vi "write_conditions_to_scope.vi"(0 "instrument handle":refnum<k15> caption="instrument handle in", 1 "Controls Cluster In":T4={"Scope Channel"="", "C1 vertical offset / V"=0.0, "C1 vertical range / V"=5.0, "C1 probe attenuation"=1.0, "C1 vertical coupling / V"=1, "C1 enabled"=TRUE, "C1 maximum input frequency / Hz"=0.0, "C1 input impedance / ohms"=0, "C2 vertical offset / V"=0.0, "C2 vertical range / V"=5.0, "C2 probe attenuation"=1.0, "C2 vertical coupling / V"=1, "C2 enabled"=TRUE, "C2 maximum input frequency / Hz"=0.0, "C2 input impedance / ohms"=0, "Enforce realtime"=TRUE, "Samples"=0, "tmax / us "=0.0, "Trigger source"="0", "Trigger slope"=0, "Trigger delay / us"=0.0} {"C1 vertical coupling / V" items=["AC", "DC", "Ground"]; "C1 input impedance / ohms" items=["1 mega ohm"=0, "50 ohms"=2]; "C2 vertical coupling / V" items=["AC", "DC", "Ground"]; "C2 input impedance / ohms" items=["1 mega ohm"=0, "50 ohms"=2]; "Samples" items=["500 S"=500, "1 kS"=1000, "5 kS"=5000, "10 kS"=10000, "100 kS"=100000, "500 kS"=500000, "1 MS"=1000000, "2.5 MS"=2500000, "5MS"=5000000, "10 MS"=10000000, "20 MS"=20000000]; "Trigger slope" items=["Positive", "Negative"]}, 11 "error in":errorcluster) -> (3 "Controls Cluster Out":T4={"Scope Channel"="", "C1 vertical offset / V"=0.0, "C1 vertical range / V"=5.0, "C1 probe attenuation"=1.0, "C1 vertical coupling / V"=1, "C1 enabled"=TRUE, "C1 maximum input frequency / Hz"=0.0, "C1 input impedance / ohms"=0, "C2 vertical offset / V"=0.0, "C2 vertical range / V"=5.0, "C2 probe attenuation"=1.0, "C2 vertical coupling / V"=1, "C2 enabled"=TRUE, "C2 maximum input frequency / Hz"=0.0, "C2 input impedance / ohms"=0, "Enforce realtime"=TRUE, "Samples"=0, "tmax / us "=0.0, "Trigger source"="0", "Trigger slope"=0, "Trigger delay / us"=0.0} {"C1 vertical coupling / V" items=["AC", "DC", "Ground"]; "C1 input impedance / ohms" items=["1 mega ohm"=0, "50 ohms"=2]; "C2 vertical coupling / V" items=["AC", "DC", "Ground"]; "C2 input impedance / ohms" items=["1 mega ohm"=0, "50 ohms"=2]; "Samples" items=["500 S"=500, "1 kS"=1000, "5 kS"=5000, "10 kS"=10000, "100 kS"=100000, "500 kS"=500000, "1 MS"=1000000, "2.5 MS"=2500000, "5MS"=5000000, "10 MS"=10000000, "20 MS"=20000000]; "Trigger slope" items=["Positive", "Negative"]}, 4 "instrument handle out":refnum<k15>, 15 "error out":errorcluster)   [LabVIEW 2023]
uses:
  <instrlib>/niScope/Controls/niScope vertical coupling.ctl
  <instrlib>/niScope/Controls/niScope trigger source.ctl
  <instrlib>/niScope/Controls/niScope trigger slope.ctl
  <instrlib>/niScope/Configure/Trigger/niScope Configure Trigger Digital.vi
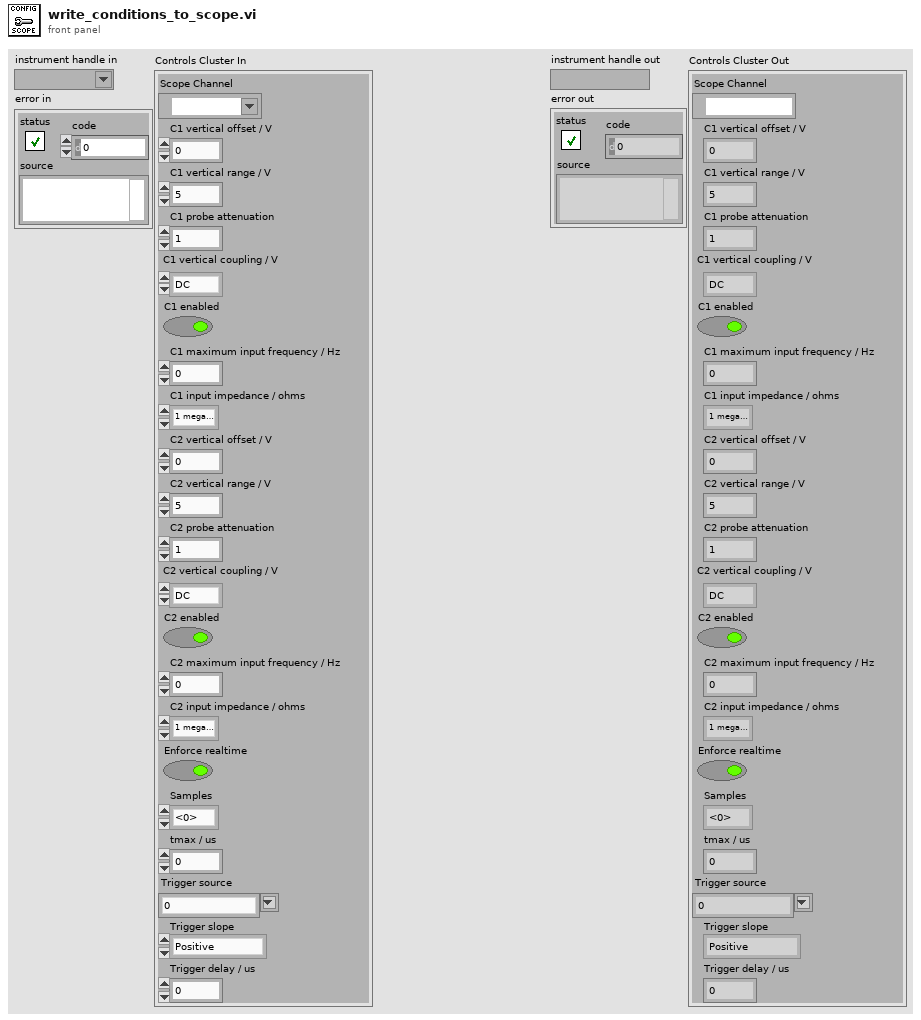
[diagram p1: front panel]
types:
  T1 = typedef "niScope vertical coupling.ctl" = i32
  T2 = typedef "niScope trigger source.ctl" = string
  T3 = typedef "niScope trigger slope.ctl" = i32
  T4 = cluster{"Scope Channel":refnum<k15>, "C1 vertical offset / V":dbl, "C1 vertical range / V":dbl, "C1 probe attenuation":dbl, "C1 vertical coupling / V":T1, "C1 enabled":bool, "C1 maximum input frequency / Hz":dbl, "C1 input impedance / ohms":u32, "C2 vertical offset / V":dbl, "C2 vertical range / V":dbl, "C2 probe attenuation":dbl, "C2 vertical coupling / V":T1, "C2 enabled":bool, "C2 maximum input frequency / Hz":dbl, "C2 input impedance / ohms":u32, "Enforce realtime":bool, "Samples":i64, "tmax / us ":dbl, "Trigger source":T2, "Trigger slope":T3, "Trigger delay / us":dbl}
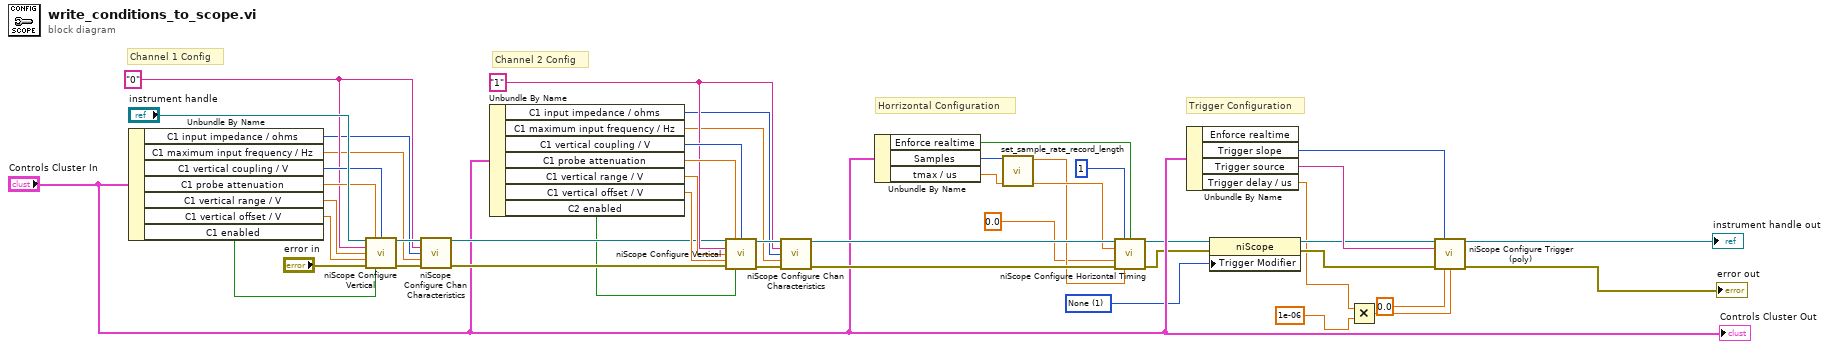
[diagram p0: block diagram]
diagram:
  w4 = 1 items=["None"=1, "Auto Trigger"=2] ("Triggering:Trigger Modifier")
  w30 = "1" ("channels")
  w39 = "0" ("channels")
  # "Trigger Configuration"
  # "Channel 2 Config"
  # "Horrizontal Configuration"
  # "Channel 1 Config"
  n1 = Unbundle By Name("Controls Cluster In") -> ("C1 input impedance / ohms"=w35:u32, "C1 maximum input frequency / Hz"=w36:dbl, "C1 vertical coupling / V"=w40:T1, "C1 probe attenuation"=w41:dbl, "C1 vertical range / V"=w38:dbl, "C1 vertical offset / V"=w37:dbl, "C1 enabled"=w12:bool)
  n2 = call <instrlib>:"niScope Configure Vertical.vi"("instrument handle"="instrument handle", "probe attenuation"=w41, "vertical coupling"=w40, "channels"=w39, "vertical range"=w38, "vertical offset"=w37, "error in"="error in", "channel enabled"=w12) -> ("instrument handle out"=w47:refnum<k15>, "error out"=w46:errorcluster)  [unwired: 6 in]
  n3 = call <instrlib>:"niScope Configure Chan Characteristics.vi"("instrument handle"=w47, "channels"=w39, "input impedance"=w35, "maximum input frequency"=w36, "error in"=w46) -> ("instrument handle out"=w25:refnum<k15>, "error out"=w24:errorcluster)  [unwired: 9 in]
  n4 = Unbundle By Name("Controls Cluster In") -> ("C1 input impedance / ohms"=w26:u32, "C1 maximum input frequency / Hz"=w27:dbl, "C1 vertical coupling / V"=w31:T1, "C1 probe attenuation"=w32:dbl, "C1 vertical range / V"=w29:dbl, "C1 vertical offset / V"=w28:dbl, "C2 enabled"=w11:bool)
  n5 = call <instrlib>:"niScope Configure Vertical.vi"("instrument handle"=w25, "probe attenuation"=w32, "vertical coupling"=w31, "channels"=w30, "vertical range"=w29, "vertical offset"=w28, "error in"=w24, "channel enabled"=w11) -> ("instrument handle out"=w34:refnum<k15>, "error out"=w33:errorcluster)  [unwired: 6 in]
  n6 = call <instrlib>:"niScope Configure Chan Characteristics.vi"("instrument handle"=w34, "channels"=w30, "input impedance"=w26, "maximum input frequency"=w27, "error in"=w33) -> ("instrument handle out"=w19:refnum<k15>, "error out"=w20:errorcluster)  [unwired: 9 in]
  n7 = Unbundle By Name("Controls Cluster In") -> ("Enforce realtime"=w23:bool, "Samples"=w22:i64, "tmax / us"=w21:dbl)
  n8 = call "set_sample_rate_record_length.vi"("t max / us"=w21, "Samples"=w22) -> ("Min sample rate"=w18:dbl, "Min record length"=w17:dbl)  [unwired: 8 in]
  n9 = call <instrlib>:"niScope Configure Horizontal Timing.vi"("instrument handle"=w19, "number of records"=1, "enforce realtime"=w23, "min sample rate"=w18, "reference position"=0.0, "error in"=w20, "min record length"=w17) -> ("instrument handle out"=w8:refnum<k15>, "error out"=w5:errorcluster)  [unwired: 7 in]
  n10 = Unbundle By Name("Controls Cluster In") -> ("Trigger slope"=w14:T3, "Trigger source"=w9:T2, "Trigger delay / us"=w2:dbl)  [unwired: 1 out]
  n11 = property on="Property Node" class="niScope"(reference=w8, error in=w5, "Trigger Modifier"=w4) -> (reference out=w7:refnum<k15>, error out=w6:errorcluster)
  n12 = Multiply(x=w2, y=1e-06) -> (x*y=w3:dbl)
  n13 = call-poly <instrlib>:"niScope Configure Trigger (poly).vi"("instrument handle"=w7, "trigger slope"=w14, "trigger source"=w9, "error in"=w6, "trigger holdoff"=0.0, "trigger delay"=w3) -> ("instrument handle out"=→"instrument handle out":refnum<k15>, "error out"=→"error out":errorcluster)  [unwired: 8 in]
  "Controls Cluster Out" <- "Controls Cluster In"
